vi "octave_open.vi"(5 "use stderr":bool, 6 "'lv_proc.dll' path":path, 7 "timeout [ms]":i32, 8 "error in":errorcluster, 10 "folder":string="c:\\octave\\bin\\", 11 "command":string="c:\\octave\\bin\\octave.exe -q") -> (0 "error out":errorcluster, 1 "initial garbage":string, 2 "version string":string, 3 "process instance handle out":u32[](array[numeric]))   [LabVIEW 2011]
doc: "Tries to creates GNU Octave process instance. Its handle is stored in global variable so its not necessary to pass it to another VIs from Octave interface library - library VIs then reads the handle from global variable automatically. Instance handle inputs/outputs are required only in case you need multiple instances of GNU Octave running at the same time.\nVI waits for console ready if timeout input is non-zero. Otherwise it only starts the process and you have to check ready state manually."
uses:
  octave_var.vi
  <vilib>/regexp/Match Regular Expression.xnode
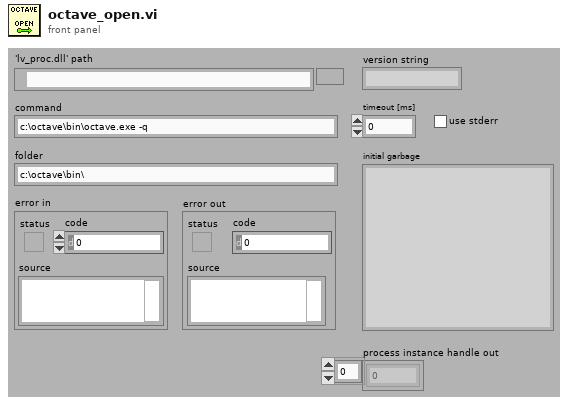
[diagram p1: front panel]
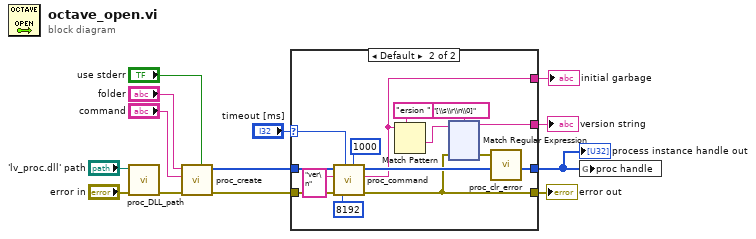
[diagram p0: block diagram]
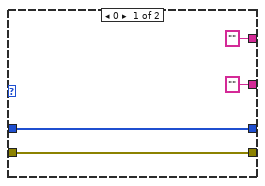
[diagram p2: hidden frame]
diagram:
  n1 = call "proc_DLL_path.vi"("error in"="error in", "path in"="'lv_proc.dll' path") -> ("error out"=w13:errorcluster)  [unwired: 8 in, 1 out]
  n2 = call "proc_create.vi"("use stderr"="use stderr", "error in"=w13, "command"="command", "folder"="folder") -> ("error out"=w5:errorcluster, "process instance handle"=w8:u32[])  [unwired: 6 in]
  n3 = case shown="Default" "timeout [ms]" {
    selector: "timeout [ms]" -> [_ w25]
    tunnel: w8 -> [w16 w31]
    tunnel: [w17 w21] -> w7
    tunnel: [w16 w28] -> w6
    tunnel: w5 -> [w17 w27]
    tunnel: ["" ("before match") w19] -> w3
    tunnel: ["" ("read buffer") w18] -> w2
    frame 0 {
    }
    frame Default {
      n4 = call "proc_command.vi"("recieve interval [ms]"=1000, "timeout [ms]"=w25, "error in"=w27, "read buffer size"=8192, "write buffer"="ver\n", "process instance handle in"=w31) -> ("error out"=w21:errorcluster, "read buffer"=w18:string, "process instance handle out"=w28:u32[])  [unwired: 1 in, 2 out]
      n5 = Match Pattern(string=w18, regular expression="ersion ") -> (after substring=w22:string)  [unwired: 1 in, 3 out]
      n6 = xnode "Match Regular Expression"("input string"=w22, "regular expression"="[\\s\\r\\n\\0]", "error in"=w21) -> ("before match"=w19:string, "error out"=w20:errorcluster)  [unwired: 3 in, 3 out]
      n7 = call "proc_clr_error.vi"("error in (no error)"=w20) -> ()  [unwired: 4 in, 1 out]
    }
  }
  "error out" <- w7
  "version string" <- w3
  "initial garbage" <- w2
  "process instance handle out" <- w6
  n8 = global write "octave_var.vi" "proc handle"(w6) -> ()
